vi "19.7-ClassicIIR-Type-CompareStepResponse.vi"() -> ()   [LabVIEW 2020]
doc: "Displays the Transfer Function of the filter selected from the front panel controls. \n\nYou can select any of the 5 IIR filter design methods (Bessel, Butterworth, Chebyshev I and II, and Elliptic) and the passband type (lowpass, highpass, bandpass, and bandstop)."
uses:
  <vilib>/Analysis/3filter.llb/Filter Passband Type.ctl
  <vilib>/Analysis/baseanly.llb/IIR Cascade Filter (DBL).vi
  <vilib>/Analysis/NI_AALBase.lvlib
panel:
  in  "Order":i32(slide)=10 scale=1.0..20.0
  out "Filtered":dbl[][](graph)
  in  "LowCutoff(3dB)":dbl=250.0 format="%#.6g"
  in  "HighCutoff(3dB)":dbl=450.0 format="%#.6g"
  out "ZoomIn":dbl[][](graph)
  in  "Type":T1
  in  "Stop":bool
  in  "Fs":dbl=1024.0 format="%#.6g"
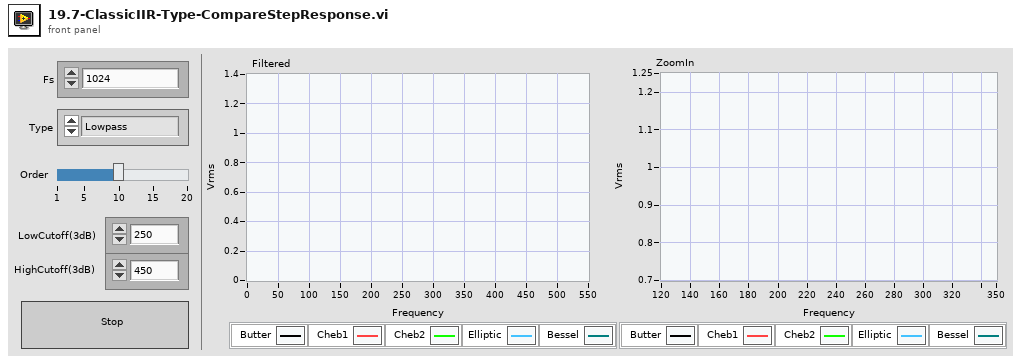
[diagram p1: front panel]
types:
  T1 = typedef "NI_AALBase.lvlib/Filter Passband Type.ctl" = enum32{"Lowpass", "Highpass", "Bandpass", "Bandstop"}
  T2 = cluster{"filter structure":enum32{"IIR 2nd Order", "IIR 4th Order"}, "Reverse Coefficients":dbl[], "Forward Coefficients":dbl[]}
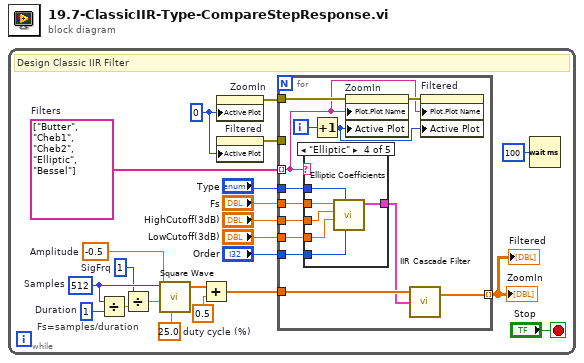
[diagram p0: block diagram]
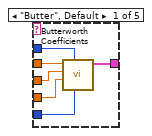
[diagram p2: hidden frame]
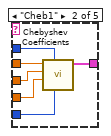
[diagram p3: hidden frame]
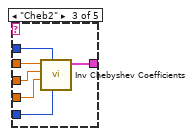
[diagram p4: hidden frame]
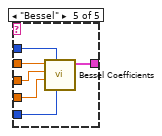
[diagram p5: hidden frame]
diagram:
  n1 = while {
    stop <- "Stop" stop-if-true
    w10 = 1  # Duration
    w7 = 1  # SigFrq
    w5 = 25.0  # duty cycle (%)
    w6 = -0.5  # Amplitude
    w9 = 512  # Samples
    w15 = string[] ["Butter", "Cheb1", "Cheb2", "Elliptic", "Bessel"]  # Filters
    w2 = u32 0 ("Active Plot")
    # "Fs=samples/duration"
    # "Design Classic IIR Filter"
    n2 = Divide(x=w9, y=w10) -> (x/y=w11:dbl)
    n3 = Divide(x=w7, y=w11) -> (x/y=w12:dbl)
    n4 = call <vilib>:"Square Wave.vi"("samples"=w9, "amplitude"=w6, "frequency"=w12, "duty cycle (%)"=w5) -> ("square wave"=w13:dbl[])  [unwired: 2 in, 2 out]
    n5 = Add(x=w13, y=0.5) -> (x+y=w4:dbl[])
    n6 = property on="ZoomIn" class="WFGraph (strict)"("Active Plot"=w2) -> (error out=w14:errorcluster)  [unwired: 2 in, 1 out]
    n7 = property on="Filtered" class="WFGraph (strict)"("Active Plot"=w2) -> (error out=w1:errorcluster)  [unwired: 2 in, 1 out]
    n8 = for {
      tunnel: "Type" -> [w35]
      tunnel: "Fs" -> [w34]
      tunnel: "HighCutoff(3dB)" -> [w33]
      tunnel: "LowCutoff(3dB)" -> [w32]
      tunnel: w15 -> [w24] mode=indexing
      tunnel: "Order" -> [w31]
      tunnel: w14 -> [w29]
      tunnel: w4 -> [w28]
      tunnel: [w26] -> w3 mode=indexing
      tunnel: w1 -> [_]
      i -> [w30]
      n9 = case shown="\"Elliptic\"" w24 {
        tunnel: w35 -> [w39 w46 w53 w59 w64]
        tunnel: w34 -> [w40 w45 w51 w57 w63]
        tunnel: [w41 w47 w52 w58 w65] -> w27
        tunnel: w33 -> [w38 w44 w50 w56 w61]
        tunnel: w32 -> [w37 w43 w49 w55 w62]
        tunnel: w31 -> [w36 w42 w48 w54 w60]
        frame "Butter", Default {
          n10 = call <vilib>:"Butterworth Coefficients.vi"("order"=w36, "filter type"=w39, "low cutoff freq: fl"=w37, "high cutoff freq: fh"=w38, "sampling freq: fs"=w40) -> ("IIR Filter Cluster"=w41:T2)  [unwired: 5 in, 1 out]
        }
        frame "Cheb1" {
          n11 = call <vilib>:"Chebyshev Coefficients.vi"("order"=w42, "filter type"=w46, "low cutoff freq: fl"=w43, "high cutoff freq: fh"=w44, "sampling freq: fs"=w45) -> ("IIR Filter Cluster"=w47:T2)  [unwired: 5 in, 1 out]
        }
        frame "Cheb2" {
          n12 = call <vilib>:"Inv Chebyshev Coefficients.vi"("order"=w48, "filter type"=w53, "low cutoff freq: fl"=w49, "high cutoff freq: fh"=w50, "sampling freq: fs"=w51) -> ("IIR Filter Cluster"=w52:T2)  [unwired: 5 in, 1 out]
        }
        frame "Elliptic" {
          n13 = call <vilib>:"Elliptic Coefficients.vi"("order"=w54, "filter type"=w59, "low cutoff freq: fl"=w55, "high cutoff freq: fh"=w56, "sampling freq: fs"=w57) -> ("IIR Filter Cluster"=w58:T2)  [unwired: 5 in, 1 out]
        }
        frame "Bessel" {
          n14 = call <vilib>:"Bessel Coefficients.vi"("order"=w60, "filter type"=w64, "low cutoff freq: fl"=w62, "high cutoff freq: fh"=w61, "sampling freq: fs"=w63) -> ("IIR Filter Cluster"=w65:T2)  [unwired: 5 in, 1 out]
        }
      }
      n15 = Increment(x=w30) -> (x+1=w23:i32)
      n16 = property on="ZoomIn" class="WFGraph (strict)"(error in=w29, "Plot.Plot Name"=w24, "Active Plot"=w23) -> (error out=w25:errorcluster)  [unwired: 1 in, 1 out]
      n17 = call-poly <vilib>:"IIR Cascade Filter.vi"("IIR Filter Cluster"=w27, "X"=w28) -> ("Filtered X"=w26:dbl[])  [unwired: 1 in, 1 out]
      n18 = property on="Filtered" class="WFGraph (strict)"(error in=w25, "Plot.Plot Name"=w24, "Active Plot"=w23) -> ()  [unwired: 1 in, 2 out]
    }
    "ZoomIn" <- w3
    "Filtered" <- w3
    n19 = Wait (ms)(milliseconds to wait=u32 100) -> ()  [unwired: 1 out]
  }
